vi "LSX Is Vel Single Axis.vi"(8 "error in (no error)":errorcluster, 9 "pdVel":dbl, 10 "lAxis":i32, 11 "lLSID":i32) -> (0 "error out":errorcluster, 1 "pdVel out":dbl, 3 "function return":i32)   [LabVIEW 2018, in "Tango.lvlib"]
doc: "TANGOAPI int TANGOCALL LSX_IsVelSingleAxis (int lLSID, int lAxis, double *pdVel);"
uses:
  Tango.lvlib
  SubVIs/Tango_DLL.dll
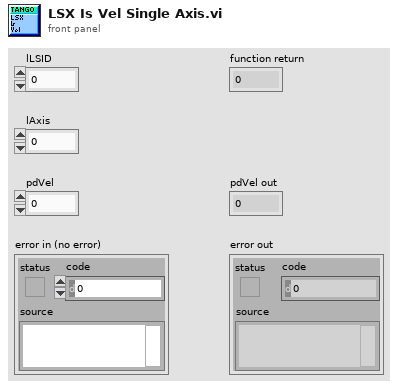
[diagram p1: front panel]
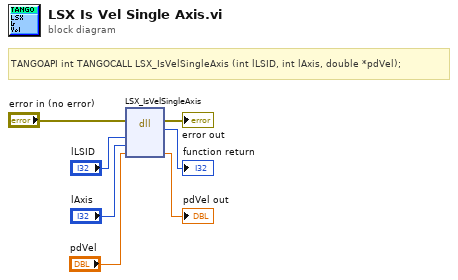
[diagram p0: block diagram]
diagram:
  # "TANGOAPI int TANGOCALL LSX_IsVelSingleAxis (int lLSID, int lAxis, double *pdVel);"
  n1 = dll-call lib="C:/Users/Familie/Documents/LabviewIX81/lib/TANGO Stage/SubVIs/Tango_DLL.*" fn="LSX_IsVelSingleAxis"(error in="error in (no error)", "lLSID"="lLSID", "lAxis"="lAxis", "pdVel"="pdVel") -> (error out=→"error out":errorcluster, →"function return":i32, "pdVel"=→"pdVel out":dbl)  [unwired: 4 in, 1 out]
